vi "FT_Get_Device_Info_Detail.vi"(0 "Device Index":u32) -> (1 "FT_Status":u32, 2 "Device Info":T1 {"Device ID" format="%x"})   [LabVIEW 2010]
uses:
  FTD2XX.dll
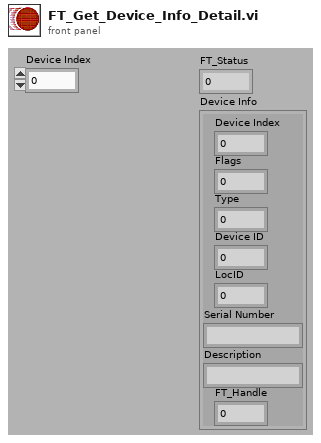
[diagram p1: front panel]
types:
  T1 = cluster{"Device Index":u32, "Flags":u32, "Type":u32, "Device ID":u32, "LocID":u32, "Serial Number":string, "Description":string, "FT_Handle":u32}
  T2 = cluster{"Device Index":u32, "Flags":u32, "Type":u32, "Device ID":u32, "LocID":i32, "Serial Number":string, "Description":string, "FT_Handle":u32}
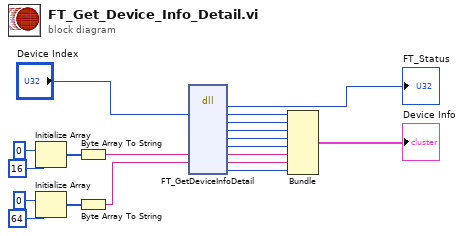
[diagram p0: block diagram]
diagram:
  n1 = Initialize Array(u8 0, 16 ("dimension size")) -> (w7:u8[])
  n2 = Initialize Array(u8 0, 64 ("dimension size")) -> (w5:u8[])
  n3 = Byte Array To String(unsigned byte array=w7) -> (string=w4:string)
  n4 = Byte Array To String(unsigned byte array=w5) -> (string=w3:string)
  n5 = dll-call lib="D:/WORK/LabView/#Avesta/D2XX_Functions_7.0/FTD2XX.dll" fn="FT_GetDeviceInfoDetail"("Device Index"="Device Index", "Serial Number"=w4, "Description"=w3) -> ("FT_Status"=→"FT_Status":u32, "Device Index"=w17:u32, "Flags"=w16:u32, "Type"=w14:u32, "Device ID"=w15:u32, "LocID"=w13:i32, "Serial Number"=w12:string, "Description"=w11:string, "FT_Handle"=w10:u32)  [unwired: 4 in, 6 out]
  n6 = Bundle("Device Index"=w17, "Flags"=w16, "Type"=w14, "Device ID"=w15, "LocID"=w13, "Serial Number"=w12, "Description"=w11, "FT_Handle"=w10) -> (→"Device Info":T2)  [unwired: 1 out]
